vi "daqio_DevTypes_FGV.vi"(6 "Dev Type in":T1, 7 "Dev Type Key":string, 8 "error in (no error)":errorcluster, 9 "Device Types in":T5[](array[typedef]), 10 "Action":T4, 11 "Device Type to return":i32=-1) -> (0 "error out":errorcluster, 1 "Dev Types out":T5[](array[typedef]), 2 "found at index":i32, 3 "added?":bool, 4 "Dev Type out":T1)   [LabVIEW 2013, in "daqio minimal.lvlib"]
doc: "This VI is a functional global variable that stores all relevant daq.io account data locally. \n\nKeeping a local device store helps with managing the device data and improves the performance of the overall system. The daq.io LabVIEW API uses this FGV to track and sync required changes that have to be performed online. This FGV should be updated whenever new channels, tags or event types need to generated. The shipping VIs that implicitly auto-create these channels, tags and events make use of this FGV.\n\nTo conserve the amount of transferred data, you can bypass the FGV and use the low level API Call Functions. Then all potential API errors, such as duplicate keys have to be managed on the client side.\n\nSee the \"Connect Device\" function to learn how this FGV can be used."
uses:
  daqio minimal.lvlib
  _typedefs/FGV_commands.ctl
  _typedefs/daqio-Channel-Type-POST-return.ctl
  _typedefs/daqio-Device.ctl
  _typedefs/daqio-Event-Type.ctl
  _typedefs/daqio-Tag-Type-POST-return.ctl
  _typedefs/daqio-Device-Type-Info-return.ctl
  _typedefs/daqio-Channels.ctl
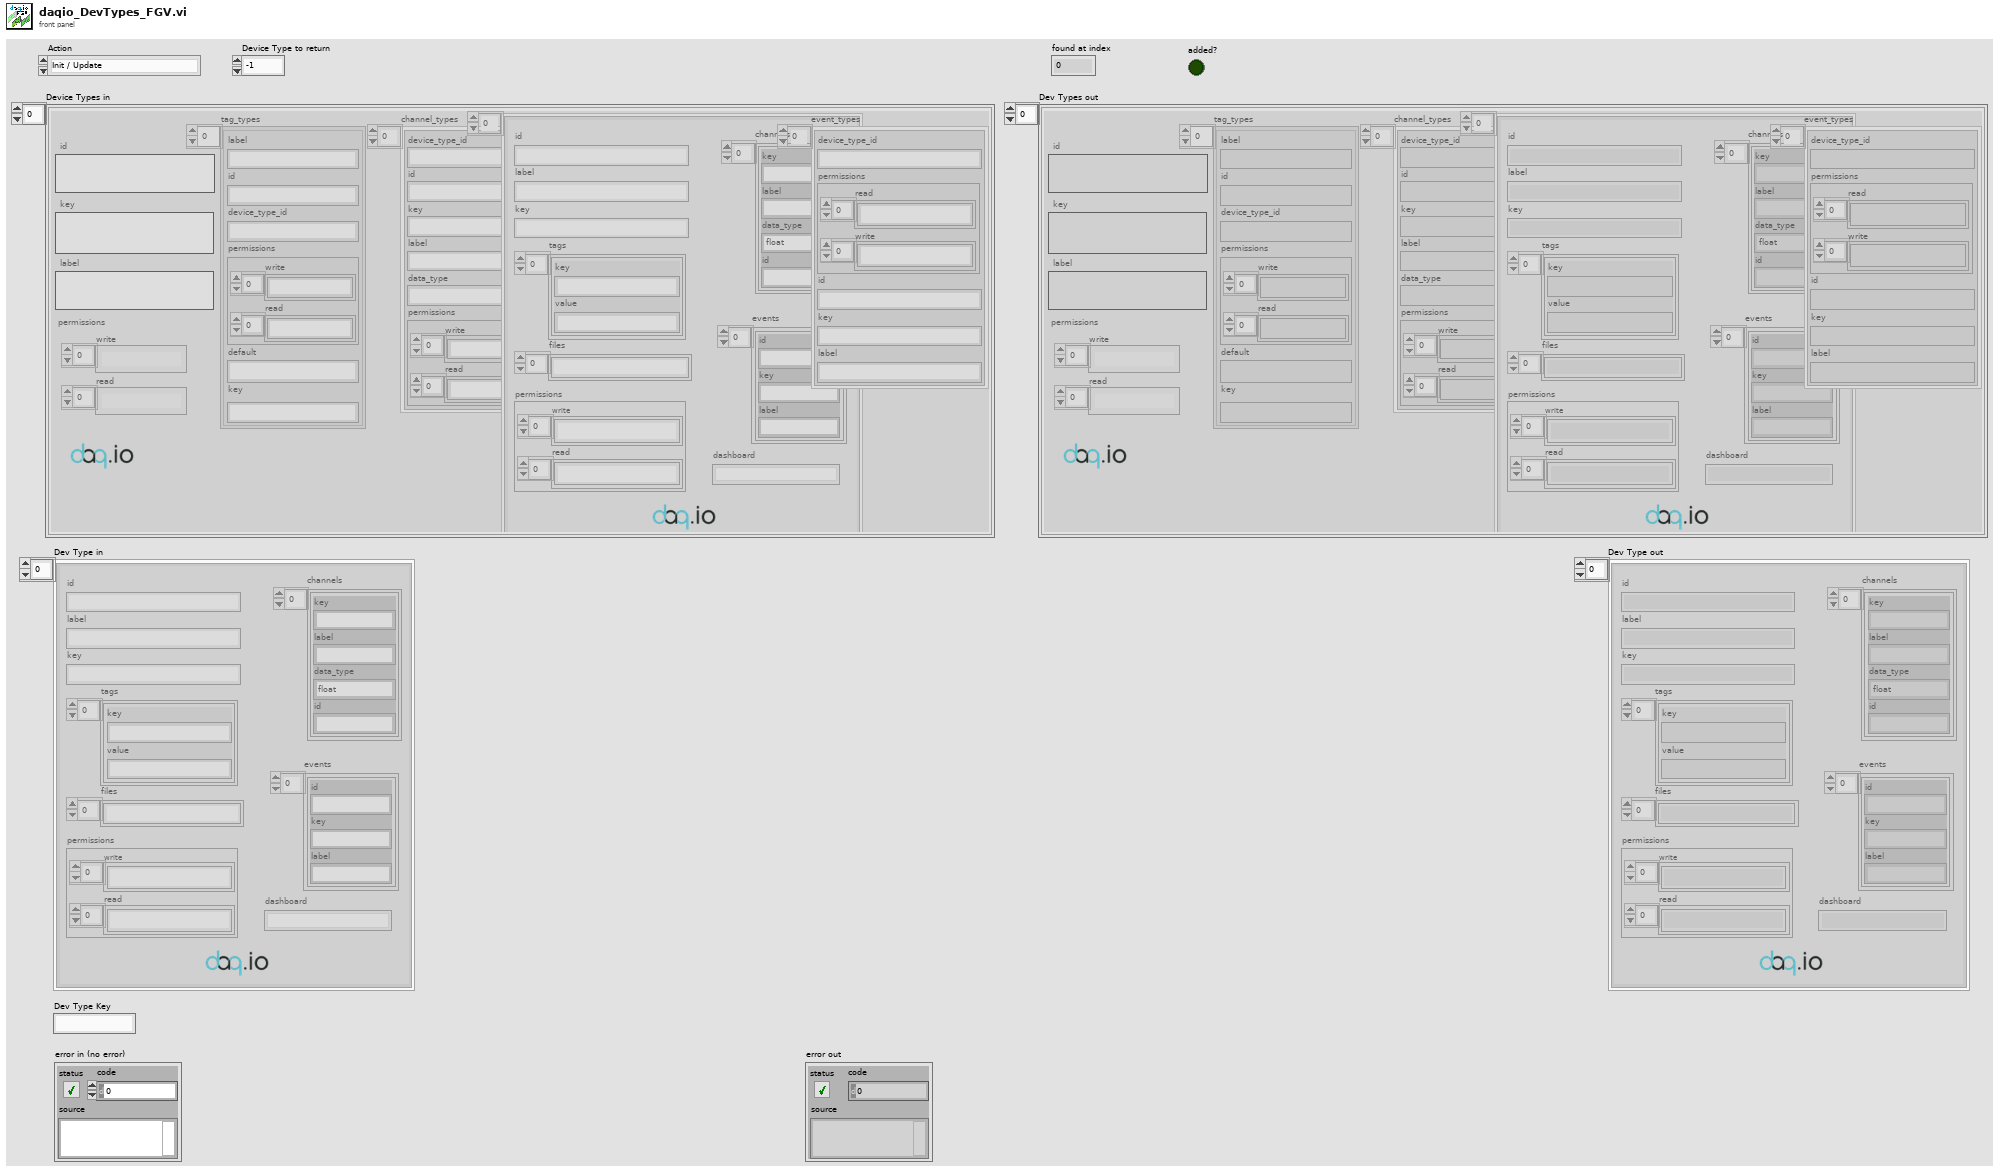
[diagram p1: front panel]
types:
  T1 = typedef "daqio minimal.lvlib/daqio-Device-Type-Info-return.ctl" = T2[]
  T2 = typedef "daqio minimal.lvlib/daqio-Device.ctl" = cluster{"id":string, "label":string, "key":string, "channels":T3[], "tags":cluster{"key":string, "value":string}[], "events":cluster{"id":string, "key":string, "label":string}[], "files":string[], "permissions":cluster{"write":string[], "read":string[]}, "dashboard":string}
  T3 = typedef "daqio minimal.lvlib/daqio-Channels.ctl" = cluster{"key":string, "label":string, "data_type":string, "id":string}
  T4 = typedef "daqio minimal.lvlib/FGV_commands.ctl" = enum16{"Init / Update", "Read From File", "Edit Item", "Find or Add Item", "Remove Item", "Delete All"}
  T5 = typedef "daqio minimal.lvlib/daqio-Device-Type-Info-return.ctl" = cluster{"channel_types":T6[], "devices":T2[], "label":string, "event_types":T7[], "key":string, "tag_types":T8[], "id":string, "permissions":cluster{"write":string[], "read":string[]}}
  T6 = typedef "daqio minimal.lvlib/daqio-Channel-Type-POST-return.ctl" = cluster{"device_type_id":string, "id":string, "key":string, "label":string, "data_type":string, "permissions":cluster{"write":string[], "read":string[]}}
  T7 = typedef "daqio minimal.lvlib/daqio-Event-Type.ctl" = cluster{"device_type_id":string, "permissions":cluster{"read":string[], "write":string[]}, "id":string, "key":string, "label":string}
  T8 = typedef "daqio minimal.lvlib/daqio-Tag-Type-POST-return.ctl" = cluster{"label":string, "id":string, "device_type_id":string, "permissions":cluster{"write":string[], "read":string[]}, "default":string, "key":string}
  T9 = enum16{"open", "replace", "create", "open or create", "replace or create", "replace or create with confirmation"}
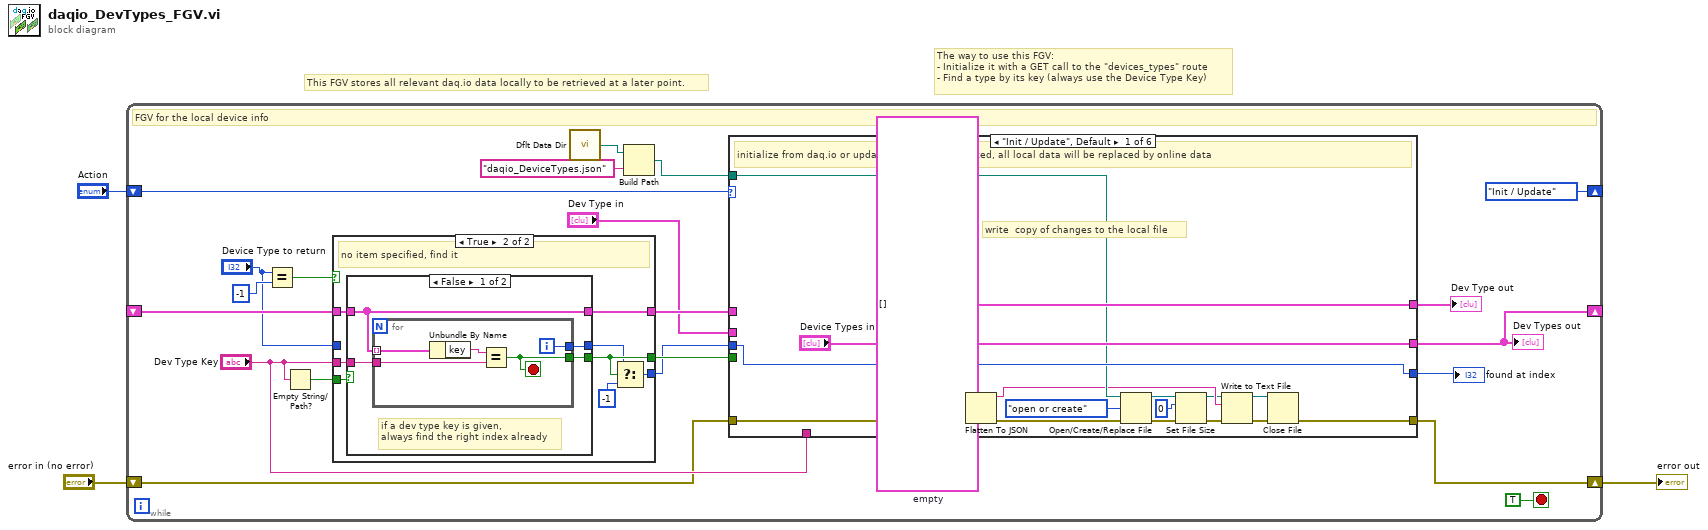
[diagram p0: block diagram]
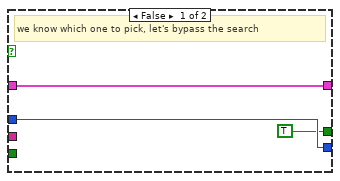
[diagram p2: hidden frame]
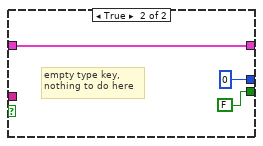
[diagram p3: hidden frame]
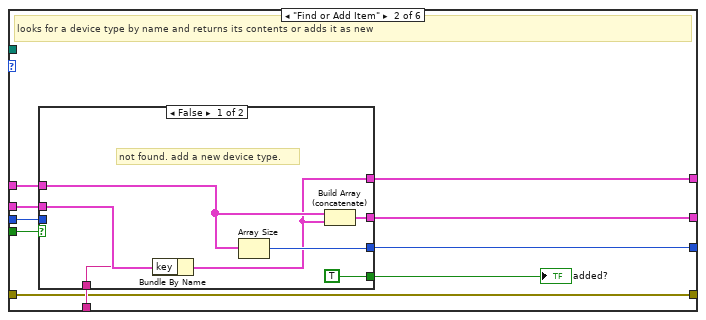
[diagram p4: hidden frame]
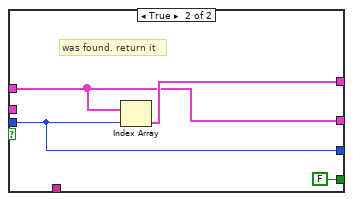
[diagram p5: hidden frame]
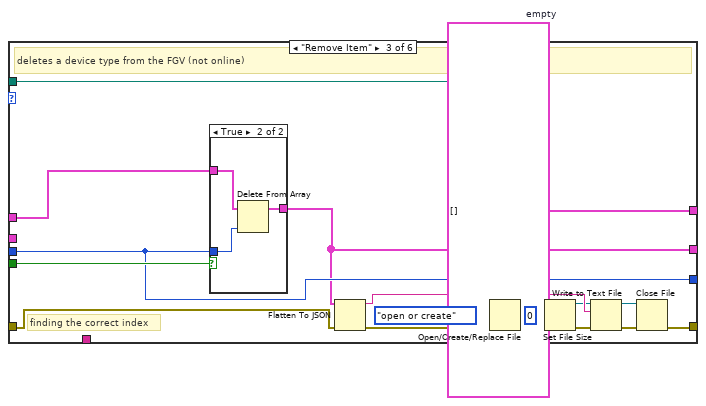
[diagram p6: hidden frame]
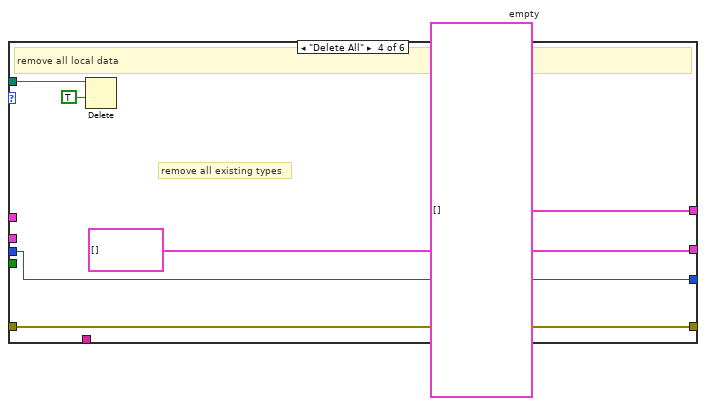
[diagram p8: hidden frame]
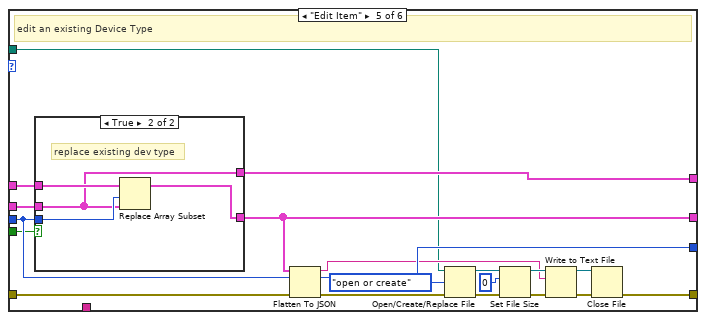
[diagram p9: hidden frame]
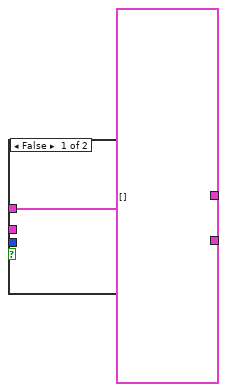
[diagram p10: hidden frame]
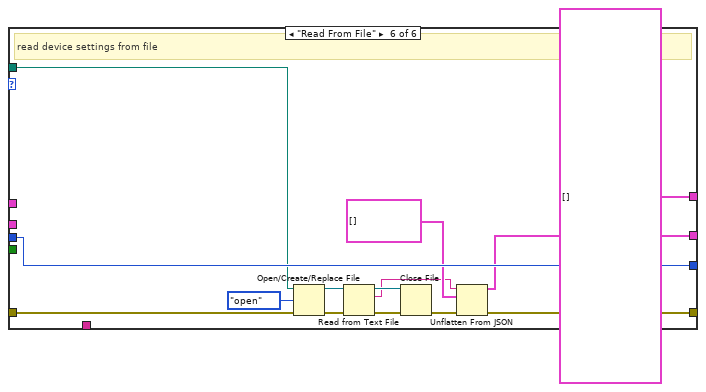
[diagram p11: hidden frame]
diagram:
  # "The way to use this FGV: \n- Initialize it with a GET call to the \"devices_types\" route\n- Find a type by its key (always use the Device Type Key)"
  # "This FGV stores all relevant daq.io data locally to be retrieved at a later point."
  n1 = while {
    shift-right: [FGV_commands."Init / Update"] -> _
    shift-left: "Action" -> [w23]
    shift-right: [w22] -> _
    shift-left: _ -> [w19]
    shift-right: [w7] -> w1
    shift-left: "error in (no error)" -> [w8]
    stop <- TRUE stop-if-true
    # "FGV for the local device info"
    n2 = Equal?(x="Device Type to return", y=-1) -> (x = y?=w11:bool)
    n3 = Empty String/Path?(string/path="Dev Type Key") -> (empty?=w20:bool)
    n4 = case shown="True" w11 {
      tunnel: w20 -> [_ w35]
      tunnel: w19 -> [w27 w34]
      tunnel: [w27 w33] -> w18
      tunnel: "Dev Type Key" -> [_ w32]
      tunnel: [TRUE w31] -> w14
      tunnel: [w26 w28] -> w9
      tunnel: "Device Type to return" -> [w26 _]
      frame False {
        # "we know which one to pick, let's bypass the search"
      }
      frame True {
        # "no item specified, find it"
        n5 = case shown="False" w35 {
          tunnel: w34 -> [w39 w47]
          tunnel: [w39 w47] -> w33
          tunnel: w32 -> [w38 _]
          tunnel: [w37 0] -> w30
          tunnel: [w36 FALSE] -> w31
          frame False {
            # "if a dev type key is given, \nalways find the right index already"
            n6 = for {
              tunnel: [w43] -> w37
              tunnel: [w42] -> w36
              tunnel: w39 -> [w41] mode=indexing
              tunnel: w38 -> [w40]
              i -> [w43]
              stop <- w42 stop-if-true
              n7 = Unbundle By Name(w41) -> ("key"=w44:string)
              n8 = Equal?(x=w44, y=w40) -> (x = y?=w42:bool)
            }
          }
          frame True {
            # "empty type key, \nnothing to do here"
          }
        }
        n9 = Select(t=w30, s=w31, f=-1) -> (s? t:f=w28:i32)
      }
    }
    n10 = call <vilib>:"Dflt Data Dir.vi"() -> ("App:Default Data Directory"=w6:path)
    n11 = Build Path(base path=w6, name or relative path="daqio_DeviceTypes.json") -> (appended path=w4:path)
    n12 = case shown="\"Init / Update\", Default" w23 {
      tunnel: ["Device Types in" w73 w86 T5[] [] ("Device Types") w115 w140] -> w22
      tunnel: w18 -> [_ w72 w102 _ w131 _]
      tunnel: w9 -> [w62 w70 w99 w110 w130 w151]
      tunnel: w14 -> [_ w71 w101 _ w129 _]
      tunnel: "Dev Type in" -> [_ w68 _ _ w128 _]
      tunnel: [w63 w69 w100 w111 w127 T1 [] ("Dev Type out 2")] -> w16
      tunnel: "Dev Type Key" -> [_ w67 _ _ _ _]
      tunnel: [w62 w65 w99 w110 w130 w151] -> w13
      tunnel: w8 -> [w60 w64 w87 w109 w116 w144]
      tunnel: [w48 w64 w88 w109 w117 w138] -> w7
      tunnel: w4 -> [w58 _ w85 w108 w113 w149]
      frame "Init / Update", Default {
        w63 = T1 []  # empty
        # "write  copy of changes to the local file"
        # "initialize from daq.io or update all values. if selected, all local data will be replaced by online data"
        n13 = Flatten To JSON(anything="Device Types in", error in (no error)=w60) -> (JSON string=w55:string, 11:w59:errorcluster)  [unwired: 1 in]
        n14 = Open/Create/Replace File(file path (use dialog)=w58, error in=w59, operation (0:open)=T9."open or create") -> (refnum out=w50:refnum<file>, error out=w49:errorcluster)  [unwired: 3 in, 1 out]
        n15 = Set File Size(4:w49, 6:i64 0 ("size (in bytes)"), 7:w50) -> (0:w52:errorcluster, 3:w53:refnum<file>)
        n16 = Write to Text File(file (use dialog)=w53, text=w55, error in=w52) -> (refnum out=w56:refnum<file>, error out=w57:errorcluster)  [unwired: 1 in, 1 out]
        n17 = Close File(refnum=w56, error in=w57) -> (error out=w48:errorcluster)  [unwired: 1 out]
      }
      frame "Find or Add Item" {
        # "looks for a device type by name and returns its contents or adds it as new"
        n18 = case shown="False" w71 {
          tunnel: [w80 w83] -> w73
          tunnel: w72 -> [w77 w83]
          tunnel: w70 -> [_ w81]
          tunnel: [w75 w84] -> w69
          tunnel: w68 -> [w79 _]
          tunnel: w67 -> [w78 _]
          tunnel: [w76 w81] -> w65
          tunnel: [TRUE FALSE] -> w66
          frame False {
            # "not found. add a new device type."
            n19 = Bundle By Name(cluster=w79, "key"=w78) -> (w75:cluster{})
            n20 = Array Size(array=w77) -> (size(s)=w76:i32)
            n21 = Build Array (concatenate)(w77, w75) -> (w80:T5[])
          }
          frame True {
            # "was found. return it"
            n22 = Index Array(array=w83, index=w81) -> (element=w84:T5)
          }
        }
        "added?" <- w66
      }
      frame "Remove Item" {
        w100 = T1 []  # empty
        # "finding the correct index"
        # "deletes a device type from the FGV (not online)"
        n23 = case shown="True" w101 {
          tunnel: w102 -> [w103 w106]
          tunnel: [w103 w105] -> w86
          tunnel: w99 -> [_ w104]
          frame False {
          }
          frame True {
            n24 = Delete From Array(array=w106, index=w104) -> (array with subset deleted=w105:T5[])  [unwired: 1 in, 1 out]
          }
        }
        n25 = Flatten To JSON(anything=w86, error in (no error)=w87) -> (JSON string=w95:string, 11:w98:errorcluster)  [unwired: 1 in]
        n26 = Open/Create/Replace File(file path (use dialog)=w85, error in=w98, operation (0:open)=T9."open or create") -> (refnum out=w90:refnum<file>, error out=w89:errorcluster)  [unwired: 3 in, 1 out]
        n27 = Set File Size(4:w89, 6:i64 0 ("size (in bytes)"), 7:w90) -> (0:w92:errorcluster, 3:w93:refnum<file>)
        n28 = Write to Text File(file (use dialog)=w93, text=w95, error in=w92) -> (refnum out=w96:refnum<file>, error out=w97:errorcluster)  [unwired: 1 in, 1 out]
        n29 = Close File(refnum=w96, error in=w97) -> (error out=w88:errorcluster)  [unwired: 1 out]
      }
      frame "Delete All" {
        w111 = T1 []  # empty
        # "remove all existing types"
        # "remove all local data"
        n30 = Delete(path (use dialog)=w108, confirm (F)=TRUE) -> ()  [unwired: 3 in, 3 out]
      }
      frame "Edit Item" {
        # "edit an existing Device Type"
        n31 = case shown="True" w129 {
          tunnel: w131 -> [w133 w137]
          tunnel: w130 -> [_ w136]
          tunnel: [w133 w135] -> w115
          tunnel: w128 -> [_ w134]
          tunnel: [T1 [] ("Dev Type in 2") w134] -> w127
          frame False {
          }
          frame True {
            # "replace existing dev type"
            n32 = Replace Array Subset(array=w137, new element=w134, index=w136) -> (w135:T5[])
          }
        }
        n33 = Flatten To JSON(anything=w115, error in (no error)=w116) -> (JSON string=w114:string, 11:w126:errorcluster)  [unwired: 1 in]
        n34 = Open/Create/Replace File(file path (use dialog)=w113, error in=w126, operation (0:open)=T9."open or create") -> (refnum out=w119:refnum<file>, error out=w118:errorcluster)  [unwired: 3 in, 1 out]
        n35 = Set File Size(4:w118, 6:i64 0 ("size (in bytes)"), 7:w119) -> (0:w121:errorcluster, 3:w122:refnum<file>)
        n36 = Write to Text File(file (use dialog)=w122, text=w114, error in=w121) -> (refnum out=w124:refnum<file>, error out=w125:errorcluster)  [unwired: 1 in, 1 out]
        n37 = Close File(refnum=w124, error in=w125) -> (error out=w117:errorcluster)  [unwired: 1 out]
      }
      frame "Read From File" {
        # "read device settings from file"
        n38 = Open/Create/Replace File(file path (use dialog)=w149, error in=w144, operation (0:open)=T9."open") -> (refnum out=w148:refnum<file>, error out=w147:errorcluster)  [unwired: 3 in, 1 out]
        n39 = Read from Text File(file (use dialog)=w148, error in=w147) -> (refnum out=w145:refnum<file>, text=w141:string, error out=w146:errorcluster)  [unwired: 2 in, 1 out]
        n40 = Close File(refnum=w145, error in=w146) -> (error out=w143:errorcluster)  [unwired: 1 out]
        n41 = Unflatten From JSON(JSON string=w141, type and defaults=T5[] [] ("Device Types in 2"), error in (no error)=w143) -> (value=w140:T5[], error out=w138:errorcluster)  [unwired: 4 in]
      }
    }
    "Dev Types out" <- w22
    "Dev Type out" <- w16
    "found at index" <- w13
  }
  "error out" <- w1
